vi "WPI_CANJaguar_SetVoltageRampRate.vi"(8 "error in (no error)":errorcluster, 10 "VoltageRampRate (V/s)":dbl, 11 "CAN Jaguar Ref":T1={"DeviceStatus"={"status"=FALSE, "code"=0, "source"=""}, "Type"=enum."PWM", "PWM"={"PWM Channel"=enum."PWM 1", "DeadBand"={"Name"="", "maxPositivePwm"=0, "minPositivePwm"=0, "centerPwm"=0, "maxNegativePwm"=0, "minNegativePwm"=0, "angularRange"=0}}, "CAN"={"Device Number"=0, "SetOutput VI Ref"=variant(enum8{"Percent VBus", "Current", "Speed", "Position", "Voltage"} enum."Percent VBus"), "GetOutput VI Ref"=variant(refnum<k1> refnum), "Enable VI Ref"=variant(dbl 12.0), "Disable VI Ref"=variant(enum8{"Percent VBus", "Speed", "Position", "Slave", "Unchanged / Invalid", "Voltage Compensation", "Current", "Motion Profile"} enum."Percent VBus"), "Data"=variant}, "Invert"=FALSE}) -> (0 "error out":errorcluster, 3 "CAN Jaguar Ref":T1={"DeviceStatus"={"status"=FALSE, "code"=0, "source"=""}, "Type"=enum."PWM", "PWM"={"PWM Channel"=enum."PWM 1", "DeadBand"={"Name"="", "maxPositivePwm"=0, "minPositivePwm"=0, "centerPwm"=0, "maxNegativePwm"=0, "minNegativePwm"=0, "angularRange"=0}}, "CAN"={"Device Number"=0, "SetOutput VI Ref"=variant(enum8{"Percent VBus", "Current", "Speed", "Position", "Voltage"} enum."Percent VBus"), "GetOutput VI Ref"=variant(refnum<k1> refnum), "Enable VI Ref"=variant(dbl 12.0), "Disable VI Ref"=variant(enum8{"Percent VBus", "Speed", "Position", "Slave", "Unchanged / Invalid", "Voltage Compensation", "Current", "Motion Profile"} enum."Percent VBus"), "Data"=variant}, "Invert"=FALSE})   [LabVIEW 2016]
doc: "Setting the <B>VoltageRampRate (V/s)</B> can be used to limit how quickly the voltage to your motor changes so that you can reduce the current required or make the changes smoother.\n\nIn <B>Percent VBus</B> mode, this is only approximate based on the <B>Max Vout</B> configuration.\n\nThis VI only applies to <B>Percent VBus</B> mode and <B>Voltage</B> mode."
uses:
  <vilib>/Rock Robotics/WPI/MotorControl/WPI_MotorControlDeviceRef.ctl
  <vilib>/Rock Robotics/WPI/MotorControl/WPI_MotorControlType.ctl
  <vilib>/Rock Robotics/SystemInterfaces/DIO/FPGA_DIOPWMChannel.ctl
  <vilib>/Rock Robotics/WPI/PWM/WPI_PWMDeadband.ctl
  <vilib>/Rock Robotics/WPI/ThirdParty/CanMotor/CAN Jaguar/SubVIs/WPI_CANJaguar_RefNumData.ctl
  <vilib>/Rock Robotics/WPI/ThirdParty/CanMotor/CAN Jaguar/SubVIs/WPI_CANJaguar_ControlMode.ctl
  <vilib>/Rock Robotics/WPI/ThirdParty/CanMotor/CAN Jaguar/SubVIs/WPI_CAN_MotorMessageIDs.ctl
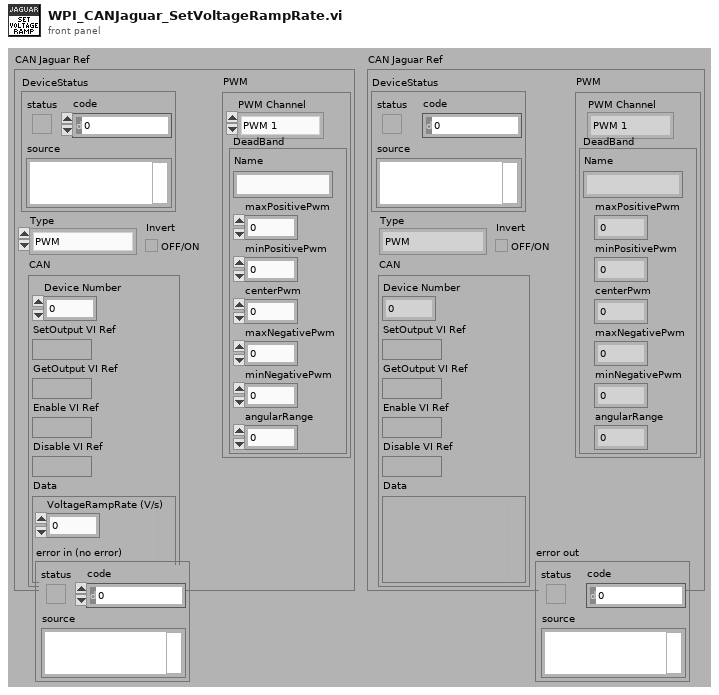
[diagram p1: front panel]
types:
  T1 = typedef "WPI_MotorControlDeviceRef.ctl" = cluster{"DeviceStatus":errorcluster, "Type":T2, "PWM":cluster{"PWM Channel":T3, "DeadBand":T4}, "CAN":cluster{"Device Number":u8, "SetOutput VI Ref":variant, "GetOutput VI Ref":variant, "Enable VI Ref":variant, "Disable VI Ref":variant, "Data":variant}, "Invert":bool}
  T2 = typedef "WPI_MotorControlType.ctl" = enum16{"PWM", "CAN"}
  T3 = typedef "FPGA_DIOPWMChannel.ctl" = enum8{"PWM 0", "PWM 1", "PWM 2", "PWM 3", "PWM 4", "PWM 5", "PWM 6", "PWM 7", "PWM 8", "PWM 9", "PWM MXP 0", "PWM MXP 1", "PWM MXP 2", "PWM MXP 3", "PWM MXP 4", "PWM MXP 5", "PWM MXP 6", "PWM MXP 7", "PWM MXP 8", "PWM MXP 9", "Invalid"}
  T4 = typedef "WPI_PWMDeadband.ctl" = cluster{"Name":string, "maxPositivePwm":i32, "minPositivePwm":i32, "centerPwm":i32, "maxNegativePwm":i32, "minNegativePwm":i32, "angularRange":u16}
  T5 = typedef "WPI_CANJaguar_RefNumData.ctl" = cluster{"CAN.Max Vout":dbl, "Control Mode":T6, "semaphore":T7}
  T6 = typedef "WPI_CANJaguar_ControlMode.ctl" = enum8{"Percent VBus", "Current", "Speed", "Position", "Voltage"}
  T7 = typedef "Semaphore RefNum" = refnum<k1>
  T8 = enum16{"big-endian, network order", "native, host order", "little-endian"}
  T9 = typedef "WPI_CAN_MotorMessageIDs.ctl" = u32
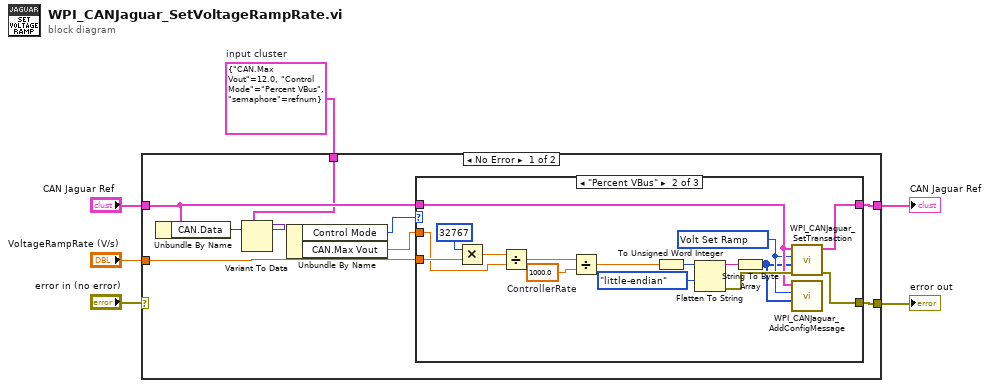
[diagram p0: block diagram]
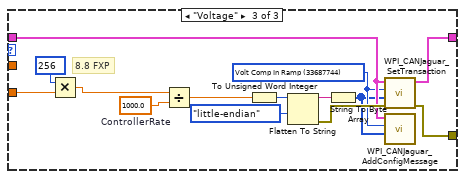
[diagram p3: hidden frame]
diagram:
  w1 = T5 {"CAN.Max Vout"=12.0, "Control Mode"=enum."Percent VBus", "semaphore"=refnum}  # input cluster
  n1 = case shown="No Error" "error in (no error)" {
    selector: "error in (no error)" -> [_ w48]
    tunnel: [w13 w48] -> w6
    tunnel: [w12 w47] -> w4
    tunnel: "CAN Jaguar Ref" -> [w14 w47]
    tunnel: "VoltageRampRate (V/s)" -> [w15 _]
    tunnel: w1 -> [w11 _]
    frame No Error {
      n2 = Unbundle By Name(w14) -> ("CAN.Data"=w10:variant)
      n3 = Variant To Data(type=w11, Variant=w10) -> (data=w9:T5)  [unwired: 1 in, 1 out]
      n4 = Unbundle By Name(w9) -> ("Control Mode"=w8:T6, "CAN.Max Vout"=w7:dbl)
      n5 = case shown="\"Percent VBus\"" w8 {
        tunnel: [_ w21 w37] -> w13
        tunnel: w15 -> [_ w28 w42]
        tunnel: w14 -> [w16 w19 w35]
        tunnel: [w16 w23 w39] -> w12
        tunnel: w7 -> [_ w20 _]
        frame Default {
        }
        frame "Percent VBus" {
          w29 = 1000.0  # ControllerRate
          w18 = T9 33685696 items=["Volt Enable"=33685504, "Volt Disable"=33685568, "Volt Set"=33685632, "Volt Set Ramp"=33685696, "Speed Enable"=33686528, "Speed Disable"=33686592, "Speed Set"=33686656, "Speed P"=33686720, "Speed I"=33686784, "Speed D"=33686848, "Speed Ref"=33686912, "Volt Comp Enable"=33687552, "Volt Comp Disable"=33687616, "Volt Comp Set"=33687680, "Volt Comp In Ramp"=33687744, "Volt Comp Comp Ramp"=33687808, "Position Enable"=33688576, "Position Disable"=33688640, "Position Set"=33688704, "Position P"=33688768, "Position I"=33688832, "Position D"=33688896, "Position Ref"=33688960, "Current Enable"=33689600, "Current Disable"=33689664, "Current Set"=33689728, "Current P"=33689792, "Current I"=33689856, "Current D"=33689920, "Status Percent VBus"=33690624, "Status VBus"=33690688, "Status Current"=33690752, "Status Temp"=33690816, "Status Position"=33690880, "Status Speed"=33690944, "Status Limit"=33691008, "Status Fault"=33691072, "Status Power"=33691136, "Status Control Mode"=33691200, "Status VOut"=33691264, "Config Num Brushes"=33692672, "Config Encoder Lines"=33692736, "Config Pot Turns"=33692800, "Config Brake Coast"=33692864, "Config Limit Mode"=33692928, "Config Limit Fwd"=33692992, "Config Limit Rev"=33693056, "Config Max VOut"=33693120, "Config Fault Time"=33693184, "Motor Ack"=33693696] ("CAN Motor Message IDs")
          n6 = Multiply(x=u32 32767 ("unsigned 16bit integer"), y=w28) -> (x*y=w26:dbl)
          n7 = Divide(x=w26, y=w20) -> (x/y=w27:dbl)
          n8 = Divide(x=w27, y=w29) -> (x/y=w24:dbl)
          n9 = To Unsigned Word Integer(number=w24) -> (unsigned 16bit integer=w30:u16)
          n10 = Flatten To String(anything=w30, byte order (0:big-endian, network order)=T8."little-endian") -> (data string=w31:string, error out=w22:errorcluster)  [unwired: 1 in, 2 out]
          n11 = String To Byte Array(string=w31) -> (unsigned byte array=w17:u8[])
          n12 = call <vilib>:"WPI_CANJaguar_SetTransaction.vi"("error in"=w22, "Data"=w17, "Message ID"=w18, "CAN Jaguar Ref"=w19) -> ("error out"=w21:errorcluster, "CAN Jaguar Ref Out"=w23:T1)  [unwired: 6 out]
          n13 = call <vilib>:"WPI_CANJaguar_AddConfigMessage.vi"("Data"=w17, "Message ID"=w18, "CAN Jaguar Ref"=w19) -> ()  [unwired: 9 in]
        }
        frame "Voltage" {
          w43 = 1000.0  # ControllerRate
          w34 = T9 33687744 items=["Volt Enable"=33685504, "Volt Disable"=33685568, "Volt Set"=33685632, "Volt Set Ramp"=33685696, "Speed Enable"=33686528, "Speed Disable"=33686592, "Speed Set"=33686656, "Speed P"=33686720, "Speed I"=33686784, "Speed D"=33686848, "Speed Ref"=33686912, "Volt Comp Enable"=33687552, "Volt Comp Disable"=33687616, "Volt Comp Set"=33687680, "Volt Comp In Ramp"=33687744, "Volt Comp Comp Ramp"=33687808, "Position Enable"=33688576, "Position Disable"=33688640, "Position Set"=33688704, "Position P"=33688768, "Position I"=33688832, "Position D"=33688896, "Position Ref"=33688960, "Current Enable"=33689600, "Current Disable"=33689664, "Current Set"=33689728, "Current P"=33689792, "Current I"=33689856, "Current D"=33689920, "Status Percent VBus"=33690624, "Status VBus"=33690688, "Status Current"=33690752, "Status Temp"=33690816, "Status Position"=33690880, "Status Speed"=33690944, "Status Limit"=33691008, "Status Fault"=33691072, "Status Power"=33691136, "Status Control Mode"=33691200, "Status VOut"=33691264, "Config Num Brushes"=33692672, "Config Encoder Lines"=33692736, "Config Pot Turns"=33692800, "Config Brake Coast"=33692864, "Config Limit Mode"=33692928, "Config Limit Fwd"=33692992, "Config Limit Rev"=33693056, "Config Max VOut"=33693120, "Config Fault Time"=33693184, "Motor Ack"=33693696] ("CAN Motor Message IDs")
          # "8.8 FXP"
          n14 = Multiply(x=u32 256 ("unsigned 16bit integer"), y=w42) -> (x*y=w36:dbl)
          n15 = Divide(x=w36, y=w43) -> (x/y=w40:dbl)
          n16 = To Unsigned Word Integer(number=w40) -> (unsigned 16bit integer=w44:u16)
          n17 = Flatten To String(anything=w44, byte order (0:big-endian, network order)=T8."little-endian") -> (data string=w45:string, error out=w38:errorcluster)  [unwired: 1 in, 2 out]
          n18 = String To Byte Array(string=w45) -> (unsigned byte array=w33:u8[])
          n19 = call <vilib>:"WPI_CANJaguar_SetTransaction.vi"("error in"=w38, "Data"=w33, "Message ID"=w34, "CAN Jaguar Ref"=w35) -> ("error out"=w37:errorcluster, "CAN Jaguar Ref Out"=w39:T1)  [unwired: 6 out]
          n20 = call <vilib>:"WPI_CANJaguar_AddConfigMessage.vi"("Data"=w33, "Message ID"=w34, "CAN Jaguar Ref"=w35) -> ()  [unwired: 9 in]
        }
      }
    }
    frame Error {
    }
  }
  "CAN Jaguar Ref" <- w4
  "error out" <- w6
